vi "RSZVB Trace Get RGB Color.vi"(0 "VISA session":refnum<visa-resource-name>, 5 "Trace Name (Trc1)":string="Trc1", 11 "error in (no error)":errorcluster {"code" format="%.0x"}) -> (3 "Red":dbl format="%^.3e", 4 "dup VISA session":refnum<visa-resource-name>, 6 "Green":dbl format="%^.3e", 8 "Blue":dbl format="%^.3e", 10 "Trace Width":i32, 14 "Trace Style":i32, 15 "error out":errorcluster {"code" format="%.0x"})   [LabVIEW 2011]
doc: "This VI returns the color of selected trace based on the Red/Green/Blue color model.\n\nRemote-control command(s):\nDISPlay:CMAP<13..28>:RGB?"
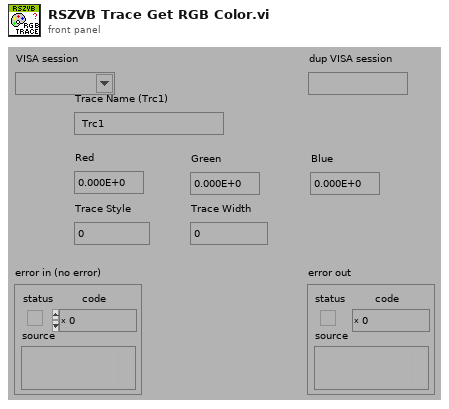
[diagram p1: front panel]
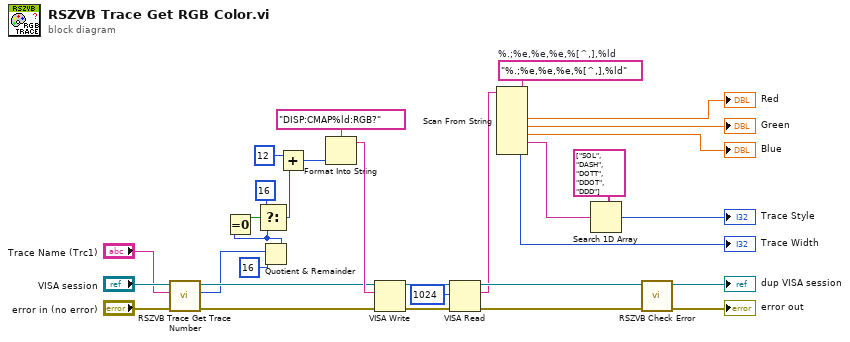
[diagram p0: block diagram]
diagram:
  w24 = "%.;%e,%e,%e,%[^,],%ld"  # %.;%e,%e,%e,%[^,],%ld
  n1 = call "RSZVB Trace Get Trace Number.vi"("error in (no error)"="error in (no error)", "Trace Name (Trc1)"="Trace Name (Trc1)", "VISA session"="VISA session") -> ("error out"=w14:errorcluster, "Trace Number"=w2:i32, "dup VISA session"=w12:refnum<visa-resource-name>)  [unwired: 6 in]
  n2 = Quotient & Remainder(x=w2, y=16) -> (x-y*floor(x/y)=w1:i32)  [unwired: 1 out]
  n3 = Equal To 0?(x=w1) -> (x = 0?=w19:bool)
  n4 = Select(t=16 ("upper limit"), s=w19, f=w1) -> (s? t:f=w17:i32)
  n5 = Add(x=12, y=w17) -> (x+y=w8:i32)
  n6 = Format Into String(format string="DISP:CMAP%ld:RGB?", w8) -> (resulting string=w13:string)  [unwired: 2 in, 1 out]
  n7 = VISA Write(VISA resource name=w12, write buffer=w13, error in (no error)=w14) -> (VISA resource name out=w26:refnum<visa-resource-name>, error out=w27:errorcluster)  [unwired: 1 out]
  n8 = VISA Read(VISA resource name=w26, byte count=u32 1024 ("byte count (0)"), error in (no error)=w27) -> (VISA resource name out=w30:refnum<visa-resource-name>, read buffer=w25:string, error out=w29:errorcluster)  [unwired: 1 out]
  n9 = Scan From String(format string=w24, input string=w25) -> (output 1=→"Red":dbl, output 2=→"Green":dbl, output 3=→"Blue":dbl, output 4=w22:string, output 5=→"Trace Width":i32)  [unwired: 7 in, 3 out]
  n10 = Search 1D Array(1D array=string[] ["SOL", "DASH", "DOTT", "DDOT", "DDD"] ("array 2"), element=w22) -> (index of element=→"Trace Style":i32)  [unwired: 1 in]
  n11 = call "RSZVB Check Error.vi"("error in (no error)"=w29, "VISA session"=w30) -> ("error out"=→"error out":errorcluster, "dup VISA session"=→"dup VISA session":refnum<visa-resource-name>)  [unwired: 8 in]
